vi "GEMM_Only(lv_gpu).vi"() -> ()   [LabVIEW 2020]
doc: "Solves the heat equation in a two-dimensional area using a Finite Element Method."
uses:
  <vilib>/addons/lvgpu/lvcuda/CUDA SGL Device Ptr/Download 2D Data.vi
  <vilib>/addons/lvgpu/lvcublas/SGEMM (aAB+bC).vi
  <vilib>/addons/lvgpu/lvcuda/CUDA SGL Device Ptr/Upload 1D Data.vi
  <vilib>/addons/lvgpu/lvcuda.lvlib
  <vilib>/addons/lvgpu/lvcublas.lvlib
  subVIs/Heat Equation Solver.lvlib
  <vilib>/addons/lvgpu/lvcuda/CUDA SGL Device Ptr/CUDA SGL Device Ptr.lvclass
  <vilib>/ptbypt/NI_PtbyPt.lvlib
panel:
  out "Heat Map":sgl[](array[numeric])
  out "time graph":dbl(graph)
  out "Error Status":errorcluster
  out "CUDA Version":string
  in  "Device ID":i32 min=0 max=0
  out "time":dbl[unit] format="%#_4p"
  in  "stop":bool
  # "GEMM based on NI's GPU Toolkit"
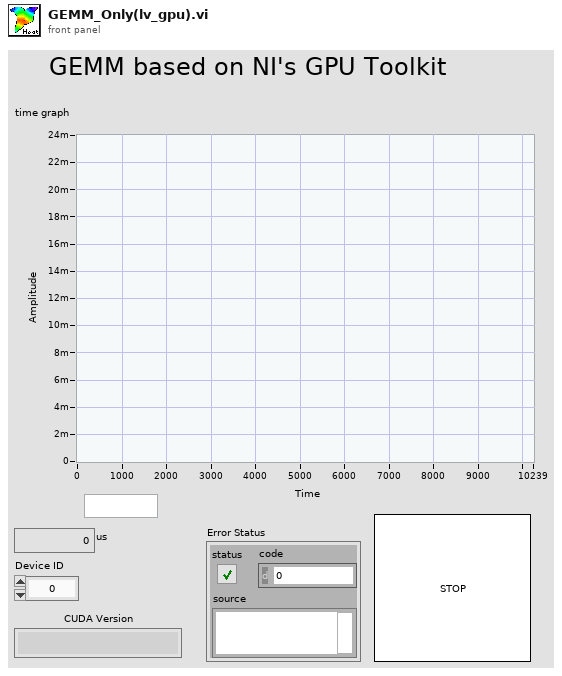
[diagram p1: front panel]
types:
  T1 = typedef "NI_Matrix.lvlib/RealMatrix.ctl" = dbl[][]
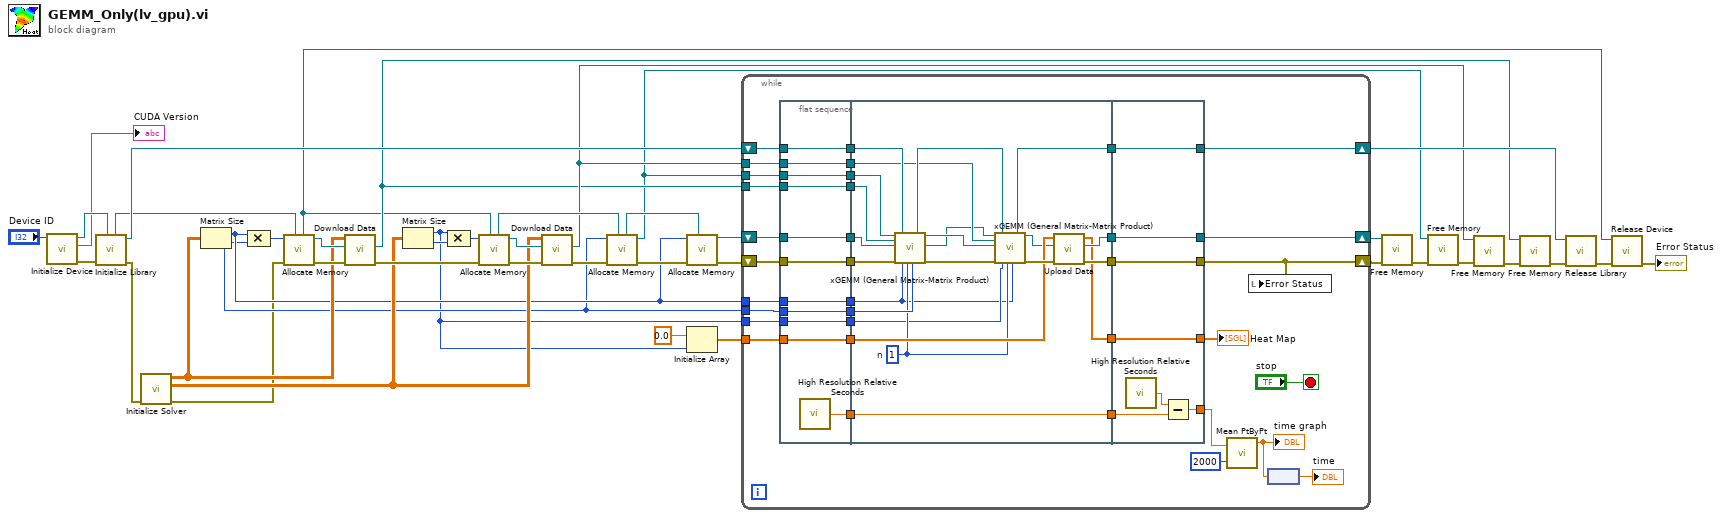
[diagram p0: block diagram]
diagram:
  n1 = call <vilib>:"Initialize Device.vi"("CUDA Device ID"="Device ID") -> ("error out"=w39:errorcluster, "CUDA Version"=→"CUDA Version":string, "CUDA Context"=w41:refnum<class "CUDA Context.lvclass">)  [unwired: 8 in]
  n2 = call <vilib>:"Initialize Library.vi"("CUDA Context in"=w41, "error in"=w39) -> ("error out"=w19:errorcluster, "CUBLAS Handle"=w42:refnum<class "CUBLAS Handle.lvclass">, "CUDA Context out"=w38:refnum<class "CUDA Context.lvclass">)  [unwired: 6 in, 1 out]
  n3 = call "Initialize Solver.vi"("error in"=w19) -> ("error out"=w2:errorcluster, "Mass"=w20:T1, "Stiffness"=w21:T1)  [unwired: 7 in, 1 out]
  n4 = Matrix Size(0:w21) -> (1:w6:i32, 2:w5:i32)
  n5 = Compound Arithmetic op=MULTIPLY(w6, w5) -> (w27:i32)
  n6 = call-poly <vilib>:"Allocate Memory.vi"("CUDA Context in"=w38, "error in"=w2, "size in elements"=w27) -> ("error out"=w25:errorcluster, "CUDA SGL Device Ptr out"=w35:refnum<class "CUDA SGL Device Ptr.lvclass">, "CUDA Context out"=w12:refnum<class "CUDA Context.lvclass">)  [unwired: 6 in]
  n7 = call-poly <vilib>:"Download Data.vi"("error in"=w25, "dst in"=w35, "src in"=w21) -> ("error out"=w24:errorcluster, "dst out"=w15:refnum<class "CUDA SGL Device Ptr.lvclass">)  [unwired: 6 in, 1 out]
  n8 = Matrix Size(0:w20) -> (1:w4:i32, 2:w26:i32)
  n9 = Compound Arithmetic op=MULTIPLY(w4, w26) -> (w36:i32)
  n10 = call-poly <vilib>:"Allocate Memory.vi"("CUDA Context in"=w12, "error in"=w24, "size in elements"=w36) -> ("error out"=w23:errorcluster, "CUDA SGL Device Ptr out"=w34:refnum<class "CUDA SGL Device Ptr.lvclass">, "CUDA Context out"=w37:refnum<class "CUDA Context.lvclass">)  [unwired: 6 in]
  n11 = call-poly <vilib>:"Download Data.vi"("error in"=w23, "dst in"=w34, "src in"=w20) -> ("error out"=w22:errorcluster, "dst out"=w16:refnum<class "CUDA SGL Device Ptr.lvclass">)  [unwired: 6 in, 1 out]
  n12 = call-poly <vilib>:"Allocate Memory.vi"("CUDA Context in"=w37, "error in"=w22, "size in elements"=w5) -> ("error out"=w11:errorcluster, "CUDA SGL Device Ptr out"=w8:refnum<class "CUDA SGL Device Ptr.lvclass">, "CUDA Context out"=w18:refnum<class "CUDA Context.lvclass">)  [unwired: 6 in]
  n13 = call-poly <vilib>:"Allocate Memory.vi"("CUDA Context in"=w18, "error in"=w11, "size in elements"=w6) -> ("error out"=w1:errorcluster, "CUDA SGL Device Ptr out"=w17:refnum<class "CUDA SGL Device Ptr.lvclass">)  [unwired: 6 in, 1 out]
  n14 = Initialize Array(sgl 0.0 ("SGL"), w4) -> (w9:sgl[])
  n15 = while {
    shift-right: [w54] -> w33
    shift-left: w42 -> [w67]
    shift-right: [w56] -> w14
    shift-left: w17 -> [w63]
    shift-right: [w55] -> w13
    shift-left: w1 -> [w61]
    tunnel: w16 -> [w71]
    tunnel: w15 -> [w70]
    tunnel: w8 -> [w65]
    tunnel: w6 -> [w51]
    tunnel: w9 -> [w59]
    tunnel: w5 -> [w49]
    tunnel: w4 -> [w47]
    stop <- "stop" stop-if-true
    n16 = flat-sequence {
      tunnel: w71 -> [w87]
      tunnel: w70 -> [w88]
      tunnel: [w88] -> w77
      tunnel: [w87] -> w76
      tunnel: [w86] -> w75
      tunnel: [w85] -> w68
      tunnel: w67 -> [w85]
      tunnel: [w84] -> w66
      tunnel: w65 -> [w84]
      tunnel: [w83] -> w64
      tunnel: w63 -> [w83]
      tunnel: [w82] -> w62
      tunnel: w61 -> [w82]
      tunnel: [w81] -> w60
      tunnel: w59 -> [w81]
      tunnel: [w80] -> w52
      tunnel: w51 -> [w80]
      tunnel: [w79] -> w50
      tunnel: w49 -> [w79]
      tunnel: [w78] -> w48
      tunnel: w47 -> [w78]
      tunnel: [w93] -> w74
      tunnel: w77 -> [w109]
      tunnel: w76 -> [w105]
      tunnel: w75 -> [w110]
      tunnel: [w110] -> w73
      tunnel: w68 -> [w108]
      tunnel: w66 -> [w103]
      tunnel: w64 -> [w104]
      tunnel: w62 -> [w102]
      tunnel: w60 -> [w98]
      tunnel: [w96] -> w58
      tunnel: [w95] -> w57
      tunnel: [w94] -> w53
      tunnel: w52 -> [w89]
      tunnel: w50 -> [w92]
      tunnel: w48 -> [w90]
      tunnel: [w117] -> w69
      tunnel: w74 -> [w117]
      tunnel: w73 -> [w116]
      tunnel: w58 -> [w113]
      tunnel: [w114] -> w56
      tunnel: w57 -> [w114]
      tunnel: [w113] -> w55
      tunnel: [w112] -> w54
      tunnel: w53 -> [w112]
      tunnel: [w111] -> w45
      frame #0 {
        n17 = call <vilib>:"High Resolution Relative Seconds.vi"() -> ("relative seconds"=w86:dbl)
      }
      frame #1 {
        w91 = 1  # n
        n18 = call-poly <vilib>:"xGEMM (General Matrix-Matrix Product).vi"("C"=w103, "A in"=w109, "B in"=w104, "error in"=w102, "CUBLAS Handle in"=w108, "m"=w89, "n"=w91, "k"=w92) -> ("CUBLAS Handle out"=w106:refnum<class "CUBLAS Handle.lvclass">, "aAB+bC"=w107:refnum<class "CUDA SGL Device Ptr.lvclass">, "B out"=w100:refnum<class "CUDA SGL Device Ptr.lvclass">, "error out"=w101:errorcluster)  [unwired: 7 in, 1 out]
        n19 = call-poly <vilib>:"xGEMM (General Matrix-Matrix Product).vi"("C"=w100, "A in"=w105, "B in"=w107, "error in"=w101, "CUBLAS Handle in"=w106, "m"=w90, "n"=w91, "k"=w89) -> ("CUBLAS Handle out"=w94:refnum<class "CUBLAS Handle.lvclass">, "aAB+bC"=w97:refnum<class "CUDA SGL Device Ptr.lvclass">, "error out"=w99:errorcluster)  [unwired: 7 in, 2 out]
        n20 = call-poly <vilib>:"Upload Data.vi"("error in"=w99, "src in"=w97, "dst in"=w98) -> ("error out"=w96:errorcluster, "src out"=w95:refnum<class "CUDA SGL Device Ptr.lvclass">, "dst out"=w93:sgl[])  [unwired: 6 in]
      }
      frame #2 {
        n21 = call <vilib>:"High Resolution Relative Seconds.vi"() -> ("relative seconds"=w115:dbl)
        n22 = Subtract(x=w115, y=w116) -> (x-y=w111:dbl)
      }
    }
    n23 = call <vilib>:"Mean PtByPt.vi"("x"=w45, "sample length"=2000) -> ("mean"=w44:dbl)  [unwired: 2 in, 1 out]
    "time graph" <- w44
    n24 = local write "Error Status"(w55) -> ()
    n25 = node(w44) -> (→"time":dbl[unit])
    "Heat Map" <- w69
  }
  n26 = call-poly <vilib>:"Free Memory.vi"("error in"=w13, "CUDA SGL Device Ptr in"=w14) -> ("error out"=w28:errorcluster)  [unwired: 9 in]
  n27 = call-poly <vilib>:"Free Memory.vi"("error in"=w28, "CUDA SGL Device Ptr in"=w8) -> ("error out"=w29:errorcluster)  [unwired: 9 in]
  n28 = call-poly <vilib>:"Free Memory.vi"("error in"=w29, "CUDA SGL Device Ptr in"=w16) -> ("error out"=w30:errorcluster)  [unwired: 9 in]
  n29 = call-poly <vilib>:"Free Memory.vi"("error in"=w30, "CUDA SGL Device Ptr in"=w15) -> ("error out"=w31:errorcluster)  [unwired: 9 in]
  n30 = call <vilib>:"Release Library.vi"("error in"=w31, "CUBLAS Handle"=w33) -> ("error out"=w32:errorcluster)  [unwired: 9 in]
  n31 = call <vilib>:"Release Device.vi"("error in"=w32, "CUDA Context in"=w12) -> ("error out"=→"Error Status":errorcluster)  [unwired: 9 in]
